vi "T7MOD_Write_with_Readback_UINT16_Register.vi"(6 "Timeout":u32=1000, 7 "UINT16 to Write":u16, 8 "error in":errorcluster, 9 "LabJack UINT16 Register":i32=55110, 10 "Remote Port":u16=502, 11 "Remote IP Address":string="192.168.1.15") -> (0 "error out":errorcluster, 1 "Written At":timestamp, 3 "nIter":i32)   [LabVIEW 2022 SP3]
panel:
  # "Input"
  # "TCP Parameters"
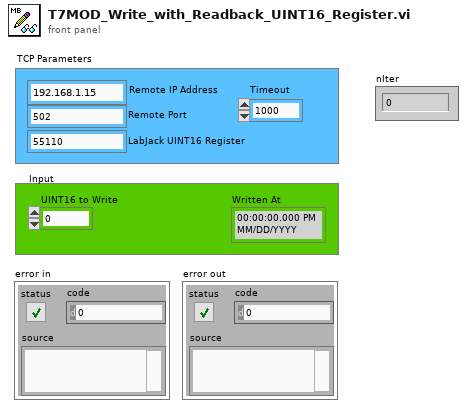
[diagram p1: front panel]
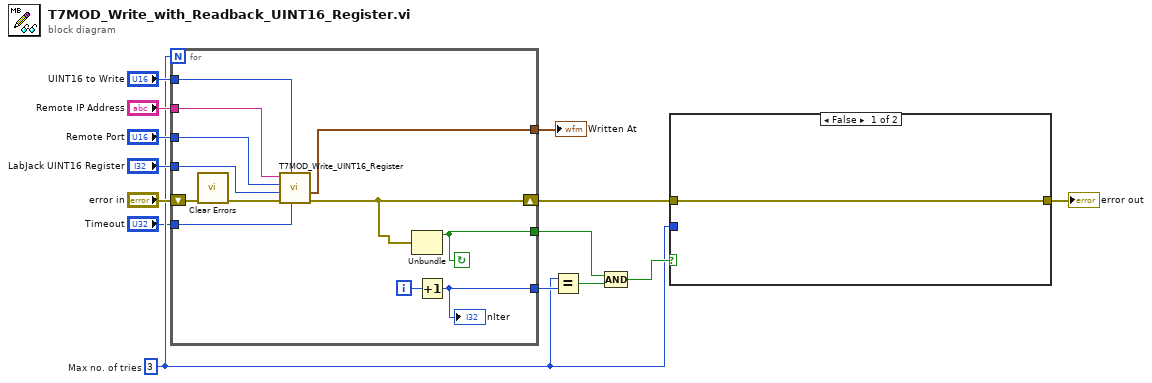
[diagram p0: block diagram]
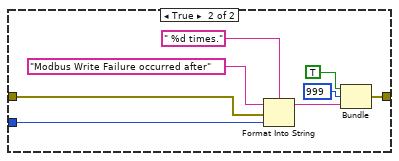
[diagram p2: hidden frame]
diagram:
  w6 = 3  # Max no. of tries
  n1 = for {
    N: w6 -> [_]
    tunnel: "Remote IP Address" -> [w26]
    shift-right: [w16] -> w4
    shift-left: "error in" -> [w18]
    tunnel: "Remote Port" -> [w25]
    tunnel: "LabJack UINT16 Register" -> [w24]
    tunnel: "UINT16 to Write" -> [w23]
    tunnel: [w20] -> w9
    tunnel: "Timeout" -> [w21]
    tunnel: [w15] -> w2
    tunnel: [w19] -> w1
    i -> [w22]
    stop <- w15 continue-if-true
    n2 = call <vilib>:"Clear Errors.vi"("error in (no error)"=w18) -> ("error out"=w17:errorcluster)  [unwired: 5 in, 1 out]
    n3 = call "T7MOD_Write_UINT16_Register.vi"("Timeout"=w21, "UINT16 to Write"=w23, "error in"=w17, "LabJack UINT16 Register"=w24, "Remote Port"=w25, "Remote IP Address"=w26) -> ("error out"=w16:errorcluster, "Written At"=w19:timestamp)  [unwired: 4 in]
    n4 = Unbundle(w16) -> ("status"=w15:bool)  [unwired: 2 out]
    n5 = Increment(x=w22) -> (x+1=w20:i32)
    "nIter" <- w20
  }
  "Written At" <- w1
  n6 = Equal?(x=w6, y=w9) -> (x = y?=w8:bool)
  n7 = Compound Arithmetic op=AND(w2, w8) -> (w7:bool)
  n8 = case shown="False" w7 {
    tunnel: w6 -> [_ w35]
    tunnel: w4 -> [w27 w32]
    tunnel: [w27 w28] -> w3
    frame False {
    }
    frame True {
      n9 = Format Into String(format string=" %d times.", initial string="Modbus Write Failure occurred after", error in=w32, w35) -> (resulting string=w29:string)  [unwired: 1 out]
      n10 = Bundle("status"=TRUE, "code"=999, w29) -> (w28:cluster{"status":bool, "code":i32, string})  [unwired: 1 in]
    }
  }
  "error out" <- w3
